vi "T7_Write_UINT32_Register.vi"(8 "UINT32 to Write":u32, 9 "LabJack UINT32 Register":i32=55120, 10 "Remote Port":u16=502, 11 "Remote IP Address":string="192.168.1.15") -> ()   [LabVIEW 2014]
uses:
  Serial Link Layer/NI_Modbus_Cleaned/NI Modbus121Clean.llb/MB Ethernet Master Query Write Multiple Registers (poly).vi
panel:
  # "MB Ethernet Example Master.vi\n\nInstructions\n1.Use Kipling to find your devices IP address & modify the\n\"Remote IP Addres\"\n2. Run this VI\n3. Change value of \"UINT32 to Write\" & press \"Write Data\""
  # "TCP Parameters"
  # "Test Write & Read of TEST_UINT32 Register"
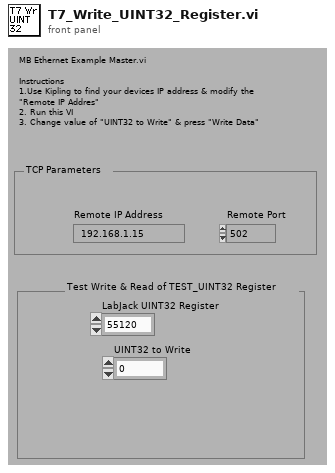
[diagram p1: front panel]
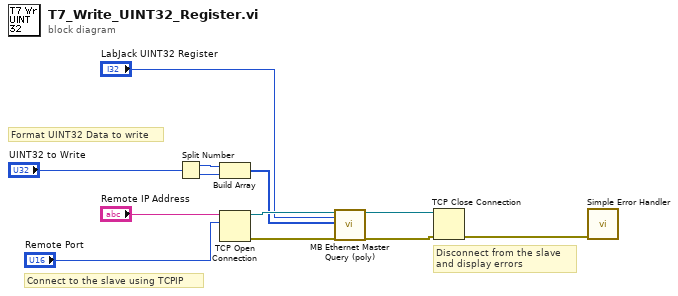
[diagram p0: block diagram]
diagram:
  # "Format UINT32 Data to write"
  # "Disconnect from the slave\nand display errors"
  # "Connect to the slave using TCPIP"
  n1 = Split Number(x="UINT32 to Write") -> (hi(x)=w3:u16, lo(x)=w1:u16)
  n2 = Build Array(w3, w1) -> (w2:u16[])
  n3 = TCP Open Connection(address="Remote IP Address", remote port or service name="Remote Port") -> (connection ID=w10:refnum<k5>, error out=w9:errorcluster)  [unwired: 3 in]
  n4 = call-poly "MB Ethernet Master Query (poly).vi"("TCP Connection Refnum in"=w10, "Starting Address"="LabJack UINT32 Register", "Registers"=w2, "error in"=w9) -> ("TCP Connection Refnum (dup)"=w6:refnum<k5>, "error out"=w7:errorcluster)  [unwired: 13 in, 1 out]
  n5 = TCP Close Connection(connection ID=w6, error in (no error)=w7) -> (error out=w8:errorcluster)  [unwired: 2 out]
  n6 = call <vilib>:"Simple Error Handler.vi"("error in (no error)"=w8) -> ()  [unwired: 1 in, 8 out]
